vi "视觉模块做视频播放.vi"() -> ()   [LabVIEW 2013]
panel:
  out "Image":T1(plugin-control)
  in  "AVI路径":path
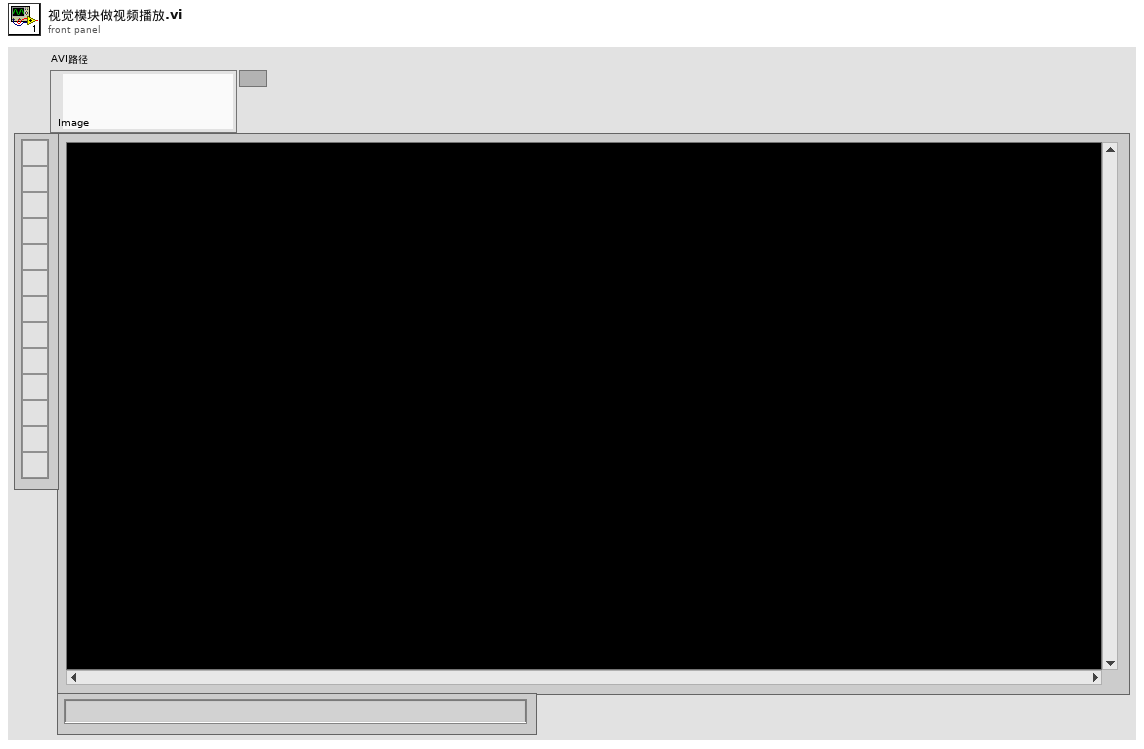
[diagram p1: front panel]
types:
  T1 = typedef "IMAQ Image.ctl" = refnum<image>
  T2 = typedef "Image Type" = u32
  T3 = typedef "IMAQ AVI2 Refnum.ctl" = refnum<k20>
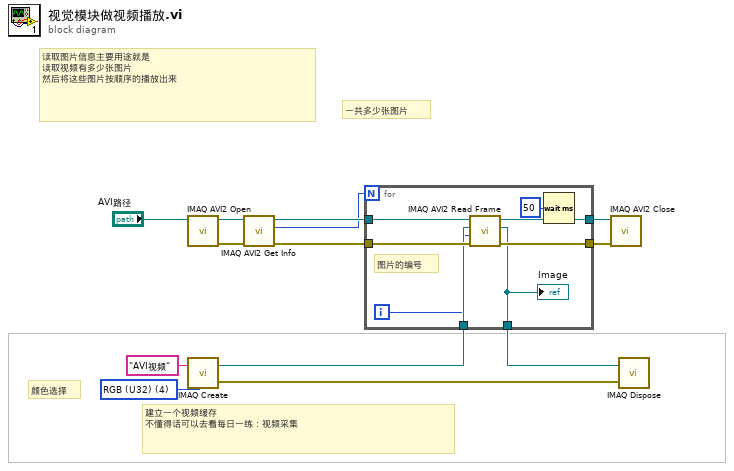
[diagram p0: block diagram]
diagram:
  w1 = T2 4 items=["Grayscale (U8)", "Grayscale (I16)", "Grayscale (SGL)", "Complex (CSG)", "RGB (U32)", "HSL (U32)", "RGB (U64)", "Grayscale (U16)"] ("Image Type")
  # "颜色选择"
  # "一共多少张图片"
  # "读取图片信息主要用途就是\n读取视频有多少张图片\n然后将这些图片按顺序的播放出来"
  # "建立一个视频缓存\n不懂得话可以去看每日一练：视频采集"
  n1 = call "IMAQ AVI2 Open"("AVI File Path"="AVI路径") -> ("error out"=w8:errorcluster, "AVI Refnum"=w13:T3)  [unwired: 9 in]
  n2 = call "IMAQ Create"("Image Name"="AVI视频", "Image Type"=w1) -> ("New Image"=w5:T1, "error out"=w6:errorcluster)  [unwired: 3 in]
  n3 = call "IMAQ AVI2 Get Info"("error in (no error)"=w8, "AVI Refnum"=w13) -> ("error out"=w9:errorcluster, "Number of Frames"=w2:u32, "AVI Refnum (duplicate)"=w12:T3)  [unwired: 5 in, 2 out]
  n4 = for {
    N: w2 -> [_]
    tunnel: w12 -> [w21]
    tunnel: [w20] -> w11
    tunnel: [w19] -> w10
    tunnel: w9 -> [w18]
    tunnel: w5 -> [w17]
    tunnel: [w16] -> w4
    i -> [w15]
    # "图片的编号"
    n5 = call "IMAQ AVI2 Read Frame"("error in (no error)"=w18, "Frame Number"=w15, "Image"=w17, "AVI Refnum"=w21) -> ("error out"=w19:errorcluster, "Image Out"=w16:T1, "AVI Refnum (duplicate)"=w20:T3)  [unwired: 5 in]
    "Image" <- w16
    n6 = Wait (ms)(milliseconds to wait=u32 50 ("等待时间（毫秒）")) -> ()  [unwired: 1 out]
  }
  n7 = call "IMAQ AVI2 Close"("error in (no error)"=w10, "AVI Refnum"=w11) -> ()  [unwired: 9 in, 1 out]
  n8 = call "IMAQ Dispose"("Image"=w4, "error in (no error)"=w6) -> ()  [unwired: 4 in, 1 out]
